vi "Test Function Path.vi"(6 "Force Built? (F)":bool, 8 "Object Type (Test Config)":T1, 9 "Object Name (\"\")":string) -> (0 "Built App?":bool, 1 "Object Path":path)   [LabVIEW 2011]
uses:
  Test Function.ctl
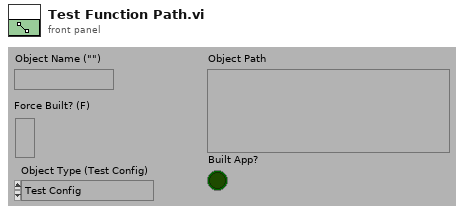
[diagram p1: front panel]
types:
  T1 = typedef "Test Function.ctl" = enum16{"Test Config", "Test Storage", "Test Pre-Process", "Unflatten Test Parameters", "Flatten Test Parameters"}
  T2 = enum32{"invalid app kind", "Development System", "Run Time System", "Student Edition", "Embedded LabVIEW", "Evaluation", "Custom"}
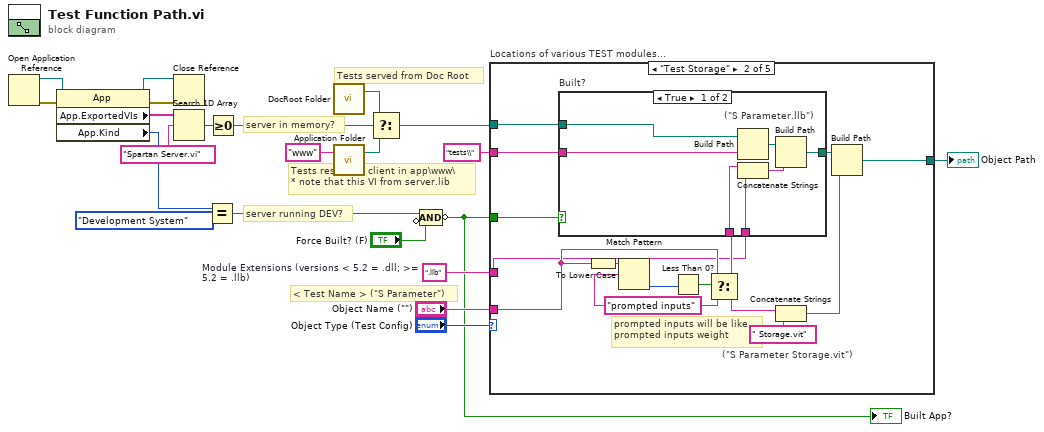
[diagram p0: block diagram]
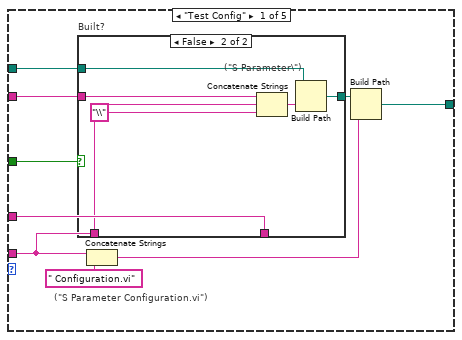
[diagram p2: hidden frame]
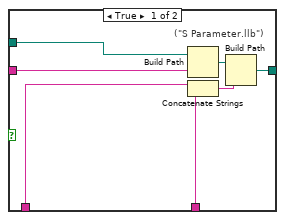
[diagram p3: hidden frame]
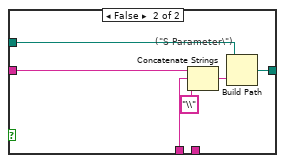
[diagram p4: hidden frame]
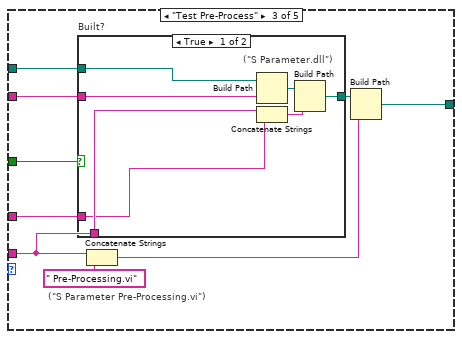
[diagram p5: hidden frame]
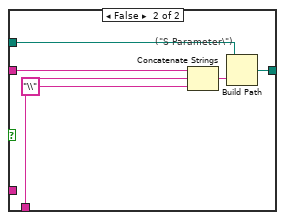
[diagram p6: hidden frame]
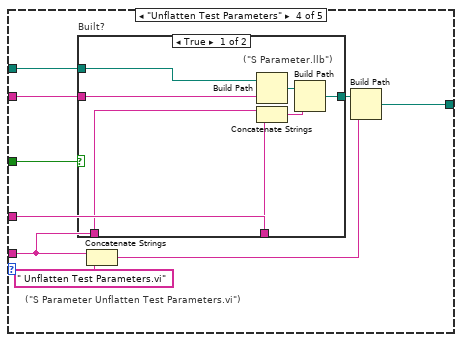
[diagram p7: hidden frame]
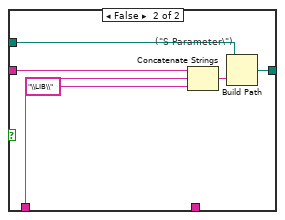
[diagram p8: hidden frame]
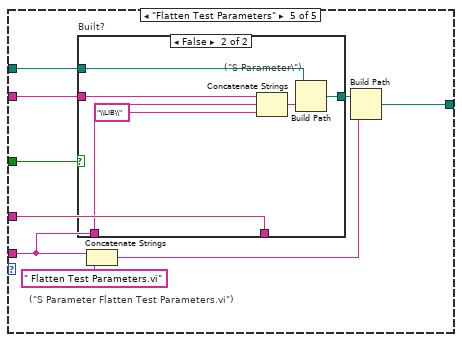
[diagram p9: hidden frame]
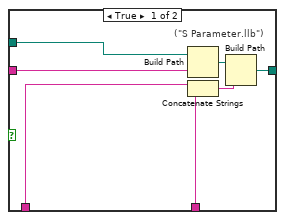
[diagram p10: hidden frame]
diagram:
  w19 = ".llb"  # Module Extensions (versions < 5.2 = .dll; >= 5.2 = .llb)
  # "server running DEV?"
  # "Tests reside on client in app\\www\\\n* note that this VI from server.lib"
  # "Tests served from Doc Root"
  # "< Test Name > (\"S Parameter\")"
  # "server in memory?"
  n1 = Open Application Reference() -> (0:w5:errorcluster, 3:w4:refnum<vi>)  [unwired: 4 in]
  n2 = property class="App"(reference=w4, error in=w5) -> (reference out=w7:refnum<vi>, error out=w6:errorcluster, "App.ExportedVIs"=w8:string[], "App.Kind"=w2:T2)
  n3 = Close Reference(reference=w7, error in (no error)=w6) -> ()  [unwired: 1 out]
  n4 = Search 1D Array(1D array=w8, element="Spartan Server.vi" ("y")) -> (index of element=w9:i32)  [unwired: 1 out]
  n5 = Equal?(x=w2, y=T2."Development System" ("Application:Kind")) -> (x = y?=w12:bool)
  n6 = Greater Or Equal To 0?(x=w9) -> (x >= 0?=w3:bool)
  n7 = call "DocRoot Folder.vi"() -> ("DocumentRoot Folder"=w18:path)  [unwired: 3 in]
  n8 = call "Application Folder.vi"("Relative Path (\"\" - Folder)"="www" ("name or relative path")) -> ("Application Folder"=w16:path)  [unwired: 2 in]
  n9 = Select(t=w18, s=w3, f=w16) -> (s? t:f=w14:path)
  n10 = Compound Arithmetic op=AND(w12, invert "Force Built? (F)") -> (invert w13:bool)
  "Built App?" <- w13
  n11 = case "Locations of various TEST modules..." shown="\"Test Storage\"" "Object Type (Test Config)" {
    tunnel: "Object Name (\"\")" -> [w27 w49 w76 w99 w121]
    tunnel: w13 -> [w26 w54 w75 w101 w120]
    tunnel: [w28 w55 w77 w102 w119] -> w20
    tunnel: w19 -> [w25 w47 w74 w96 w118]
    tunnel: "tests\\" -> [w24 w46 w73 w95 w117]
    tunnel: w14 -> [w23 w45 w72 w94 w116]
    frame "Test Config" {
      # "(\"S Parameter Configuration.vi\")"
      n12 = case "Built?" shown="False" w26 {
        tunnel: [w38 w44] -> w31
        tunnel: w27 -> [w36 w43]
        tunnel: w23 -> [w35 w39]
        tunnel: w24 -> [w34 w40]
        tunnel: w25 -> [w32 _]
        frame True {
          # "(\"S Parameter.llb\")"
          n13 = Build Path(base path=w35, name or relative path=w34) -> (appended path=w33:path)
          n14 = Concatenate Strings(w36, w32) -> (w37:string)
          n15 = Build Path(base path=w33, name or relative path=w37) -> (appended path=w38:path)
        }
        frame False {
          # "(\"S Parameter\\\")"
          n16 = Concatenate Strings(w40, w43, "\\") -> (w41:string)
          n17 = Build Path(base path=w39, name or relative path=w41) -> (appended path=w44:path)
        }
      }
      n18 = Concatenate Strings(w27, " Configuration.vi") -> (w29:string)
      n19 = Build Path(base path=w31, name or relative path=w29) -> (appended path=w28:path)
    }
    frame "Test Storage" {
      w50 = "prompted inputs"
      # "prompted inputs will be like\nprompted inputs weight"
      # "(\"S Parameter Storage.vit\")"
      n20 = To Lower Case(string=w49) -> (all lower case string=w53:string)
      n21 = Match Pattern(string=w53, regular expression=w50) -> (offset past match=w52:i32)  [unwired: 4 out]
      n22 = Less Than 0?(x=w52) -> (x < 0?=w51:bool)
      n23 = Select(t=w49, s=w51, f=w50) -> (s? t:f=w48:string)
      n24 = case "Built?" shown="True" w54 {
        tunnel: [w65 w71] -> w58
        tunnel: w48 -> [w63 w66]
        tunnel: w45 -> [w62 w67]
        tunnel: w46 -> [w61 w68]
        tunnel: w47 -> [w59 _]
        frame True {
          # "(\"S Parameter.llb\")"
          n25 = Build Path(base path=w62, name or relative path=w61) -> (appended path=w60:path)
          n26 = Concatenate Strings(w63, w59) -> (w64:string)
          n27 = Build Path(base path=w60, name or relative path=w64) -> (appended path=w65:path)
        }
        frame False {
          # "(\"S Parameter\\\")"
          n28 = Concatenate Strings(w68, w66, "\\") -> (w69:string)
          n29 = Build Path(base path=w67, name or relative path=w69) -> (appended path=w71:path)
        }
      }
      n30 = Concatenate Strings(w48, " Storage.vit") -> (w56:string)
      n31 = Build Path(base path=w58, name or relative path=w56) -> (appended path=w55:path)
    }
    frame "Test Pre-Process" {
      # "(\"S Parameter Pre-Processing.vi\")"
      n32 = case "Built?" shown="True" w75 {
        tunnel: [w87 w93] -> w78
        tunnel: w76 -> [w85 w92]
        tunnel: w72 -> [w84 w88]
        tunnel: w73 -> [w83 w89]
        tunnel: w74 -> [w81 _]
        frame True {
          # "(\"S Parameter.dll\")"
          n33 = Build Path(base path=w84, name or relative path=w83) -> (appended path=w82:path)
          n34 = Concatenate Strings(w85, w81) -> (w86:string)
          n35 = Build Path(base path=w82, name or relative path=w86) -> (appended path=w87:path)
        }
        frame False {
          # "(\"S Parameter\\\")"
          n36 = Concatenate Strings(w89, w92, "\\") -> (w90:string)
          n37 = Build Path(base path=w88, name or relative path=w90) -> (appended path=w93:path)
        }
      }
      n38 = Concatenate Strings(w76, " Pre-Processing.vi") -> (w80:string)
      n39 = Build Path(base path=w78, name or relative path=w80) -> (appended path=w77:path)
    }
    frame "Unflatten Test Parameters" {
      # "(\"S Parameter Unflatten Test Parameters.vi\")"
      n40 = case "Built?" shown="True" w101 {
        tunnel: [w109 w115] -> w100
        tunnel: w99 -> [w107 w114]
        tunnel: w94 -> [w106 w110]
        tunnel: w95 -> [w105 w111]
        tunnel: w96 -> [w103 _]
        frame True {
          # "(\"S Parameter.llb\")"
          n41 = Build Path(base path=w106, name or relative path=w105) -> (appended path=w104:path)
          n42 = Concatenate Strings(w107, w103) -> (w108:string)
          n43 = Build Path(base path=w104, name or relative path=w108) -> (appended path=w109:path)
        }
        frame False {
          # "(\"S Parameter\\\")"
          n44 = Concatenate Strings(w111, w114, "\\LIB\\") -> (w112:string)
          n45 = Build Path(base path=w110, name or relative path=w112) -> (appended path=w115:path)
        }
      }
      n46 = Concatenate Strings(w99, " Unflatten Test Parameters.vi") -> (w97:string)
      n47 = Build Path(base path=w100, name or relative path=w97) -> (appended path=w102:path)
    }
    frame "Flatten Test Parameters" {
      # "(\"S Parameter Flatten Test Parameters.vi\")"
      n48 = case "Built?" shown="False" w120 {
        tunnel: [w131 w137] -> w124
        tunnel: w121 -> [w129 w136]
        tunnel: w116 -> [w128 w132]
        tunnel: w117 -> [w127 w133]
        tunnel: w118 -> [w125 _]
        frame True {
          # "(\"S Parameter.llb\")"
          n49 = Build Path(base path=w128, name or relative path=w127) -> (appended path=w126:path)
          n50 = Concatenate Strings(w129, w125) -> (w130:string)
          n51 = Build Path(base path=w126, name or relative path=w130) -> (appended path=w131:path)
        }
        frame False {
          # "(\"S Parameter\\\")"
          n52 = Concatenate Strings(w133, w136, "\\LIB\\") -> (w134:string)
          n53 = Build Path(base path=w132, name or relative path=w134) -> (appended path=w137:path)
        }
      }
      n54 = Concatenate Strings(w121, " Flatten Test Parameters.vi") -> (w122:string)
      n55 = Build Path(base path=w124, name or relative path=w122) -> (appended path=w119:path)
    }
  }
  "Object Path" <- w20
